vi "OutputShooter2.vi"() -> ()   [LabVIEW 2020]
uses:
  GRNF_CTREMotor.vi
  <vilib>/Rock Robotics/WPI/ThirdParty/Phoenix-LabVIEW/Motor Controller/Get/CTRE_Phoenix_MotorController_GetVoltage.vi
  <vilib>/Rock Robotics/WPI/ThirdParty/Phoenix-LabVIEW/Motor Controller/Get/CTRE_Phoenix_MotorController_GetSelectedSensorData.vi
  refnumbers.vi
  robotconstants.vi
  sensordata.vi
  robotoutputs.vi
  <vilib>/Rock Robotics/WPI/ThirdParty/Phoenix-LabVIEW/Motor Controller/Controls/CTRE_Phoenix_MotorControl_ControlMode.ctl
  TAI_Motor.vi
  98ea3fb8-6e38-4b27-9b09-ea0ebeb37837.vi
  driverdata.vi
  b8824af5-e744-4a1c-8f85-7ad47afccb2a.vi
  f2b47ff3-4a7b-451f-be46-1db9049ccf7f.vi
  drivercommands.vi
  <vilib>/Rock Robotics/WPI/ThirdParty/Phoenix-LabVIEW/Motor Controller/Get/CTRE_Phoenix_MotorController_GetGeneralStatus.vi
  176032df-062a-4c80-a46a-f01413ab376a.vi
  <vilib>/Rock Robotics/WPI/DriverStation/WPI_DriverStationRobotMode2.ctl
panel:
  in  "Shooter Upper PID Configuration":T1={"P Gain"=0.006, "I Gain"=0.0, "D Gain"=0.0, "F Gain"=0.2, "I Zone"=200.0} {"I Zone" step=0.01; "F Gain" step=0.01; "D Gain" step=0.01; "I Gain" step=0.01; "P Gain" min=0.0 step=0.01}
  in  "Cowl PID Parameters":T2={"Kp"=0.03, "Ki"=0.0, "Kd"=0.0, "Kf (don't use)"=0.0, "I-Zone"=10.0} {"Kd" min=0.0; "Ki" min=0.0; "Kp" min=0.0}
  in  "Arbitrary Feed Forward [-1,1]":dbl=0.03
  in  "Cowl S-Curve Strength":i32=4
  in  "Cowl Acceleration (deg/s^2)":dbl=300.0
  in  "Cowl Cruise Velocity (deg/s)":dbl=60.0
  out "Cowl Position":cluster{dbl, "Interlock Output":dbl}(graph)
  out "Position":dbl
  out "Cowl Velocity":cluster{dbl}(graph)
  in  "Plot Cowl":bool
  in  "Manual Override Cowl":bool
  in  "Manual Cowl Command (deg)":dbl
  in  "Manual Shooter Upper Speed Goal (rpm)":dbl=1.5 min=0.0 max=6000.0 step=100.0
  in  "Manual Shooter Lower Speed Goal (rpm)":dbl min=0.0 max=6000.0 step=100.0
  in  "Override Shooter State Controller":bool
  out "Shooter Upper":T3(graph)
  out "Shooter Lower":T3(graph)
  in  "Plot Shooter":bool
  in  "Shooter Lower PID Configuration":T1={"P Gain"=0.005, "I Gain"=0.0, "D Gain"=0.0, "F Gain"=0.2, "I Zone"=200.0} {"I Zone" step=0.01; "F Gain" step=0.01; "D Gain" step=0.01; "I Gain" step=0.01; "P Gain" min=0.0 step=0.01}
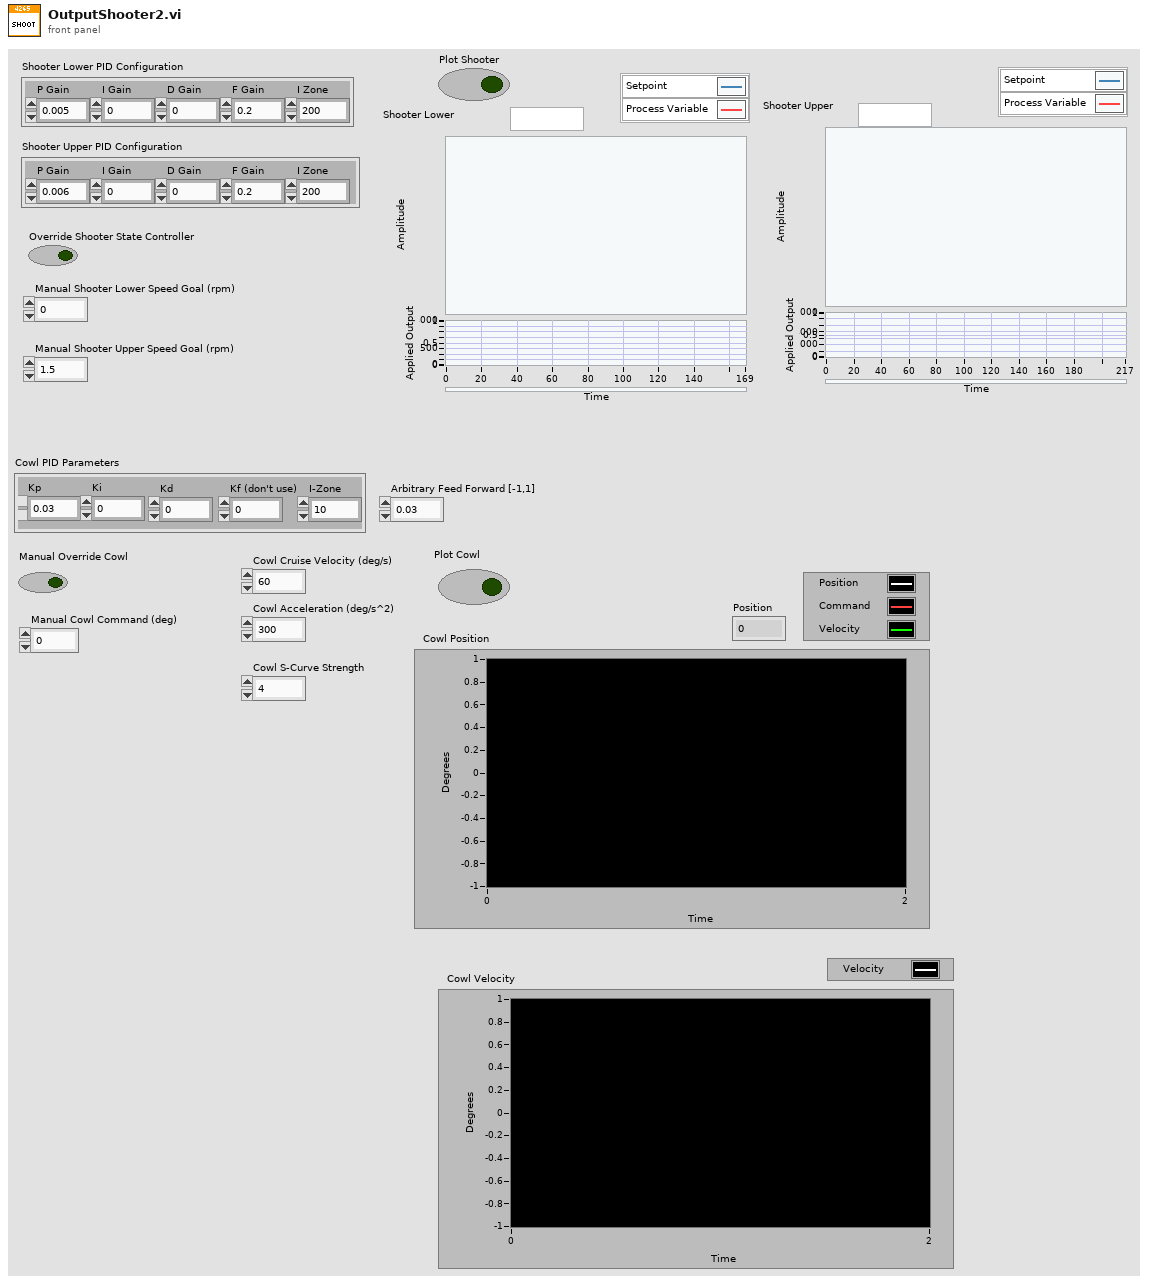
[diagram p1: front panel]
types:
  T1 = cluster{"P Gain":dbl, "I Gain":dbl, "D Gain":dbl, "F Gain":dbl, "I Zone":dbl}
  T2 = cluster{"Kp":dbl, "Ki":dbl, "Kd":dbl, "Kf (don't use)":dbl, "I-Zone":dbl}
  T3 = cluster{"Sensor Velocity":dbl, "Setpoint":dbl, "Applied Output":dbl}
  T4 = typedef "WPI_DriverStationRobotMode2.ctl" = enum16{"Autonomous Disabled", "Autonomous Enabled", "Teleop Disabled", "Teleop Enabled", "Disconnected", "Finish", "Test Disabled", "Test Enabled", "Emergency Stopped"}
  T5 = cluster{"Cowl Cruise Velocity (deg/s)":i32, "Cowl Acceleration (deg/s^2)":i32, "Cowl S-Curve Strength":i32}
  T6 = typedef "WPI_MotorControlDeviceRef.ctl" = cluster{"DeviceStatus":errorcluster, "Type":T7, "PWM":cluster{"PWM Channel":T8, "DeadBand":T9}, "CAN":cluster{"Device Number":u8, "SetOutput VI Ref":variant, "GetOutput VI Ref":variant, "Enable VI Ref":variant, "Disable VI Ref":variant, "Data":variant}, "Invert":bool, "DIO PWM":cluster{"PWM \"Enable\" Channel":T8, "DIOChannel":T10, "PWM Rate":dbl}}
  T7 = typedef "WPI_MotorControlType.ctl" = enum16{"PWM", "CAN", "DIO PWM"}
  T8 = typedef "FPGA_DIOPWMChannel.ctl" = enum8{"PWM 0", "PWM 1", "PWM 2", "PWM 3", "PWM 4", "PWM 5", "PWM 6", "PWM 7", "PWM 8", "PWM 9", "PWM MXP 0", "PWM MXP 1", "PWM MXP 2", "PWM MXP 3", "PWM MXP 4", "PWM MXP 5", "PWM MXP 6", "PWM MXP 7", "PWM MXP 8", "PWM MXP 9", "Invalid"}
  T9 = typedef "WPI_PWMDeadband.ctl" = cluster{"Name":string, "maxPositivePwm":i32, "minPositivePwm":i32, "centerPwm":i32, "maxNegativePwm":i32, "minNegativePwm":i32, "angularRange":u16}
  T10 = typedef "FPGA_DIOChannel.ctl" = enum8{"DIO 0", "DIO 1", "DIO 2", "DIO 3", "DIO 4", "DIO 5", "DIO 6", "DIO 7", "DIO 8", "DIO 9", "DIO MXP 0", "DIO MXP 1", "DIO MXP 2", "DIO MXP 3", "DIO MXP 4", "DIO MXP 5", "DIO MXP 6", "DIO MXP 7", "DIO MXP 8", "DIO MXP 9", "DIO MXP 10", "DIO MXP 11", "DIO MXP 12", "DIO MXP 13", "DIO MXP 14", "DIO MXP 15", "SPI Port CS1", "SPI Port CS2", "SPI Port CS3", "SPI Port MISO", "SPI Port MOSI", "Invalid"}
  T11 = cluster{"P Gain":bool, "I Gain":bool, "D Gain":bool, "F Gain":bool, "I Zone":bool}
  T12 = cluster{"Cowl Cruise Velocity (deg/s)":bool, "Cowl Acceleration (deg/s^2)":bool, "Cowl S-Curve Strength":bool}
  T13 = enum16{"No Changed Output", "New Normal Output", "New Testing Output"}
  T14 = cluster{"Kp":bool, "Ki":bool, "Kd":bool, "Kf (don't use)":bool, "I-Zone":bool}
  T15 = typedef "CTRE_Phoenix_MotorControl_ControlMode.ctl" = u16
  T16 = cluster{"Interlocked Output":dbl, dbl, "Percent Output":dbl}
  T17 = enum16{"DemandType_Neutral", "DemandType_AuxPID", "DemandType_ArbitraryFeedForward"}
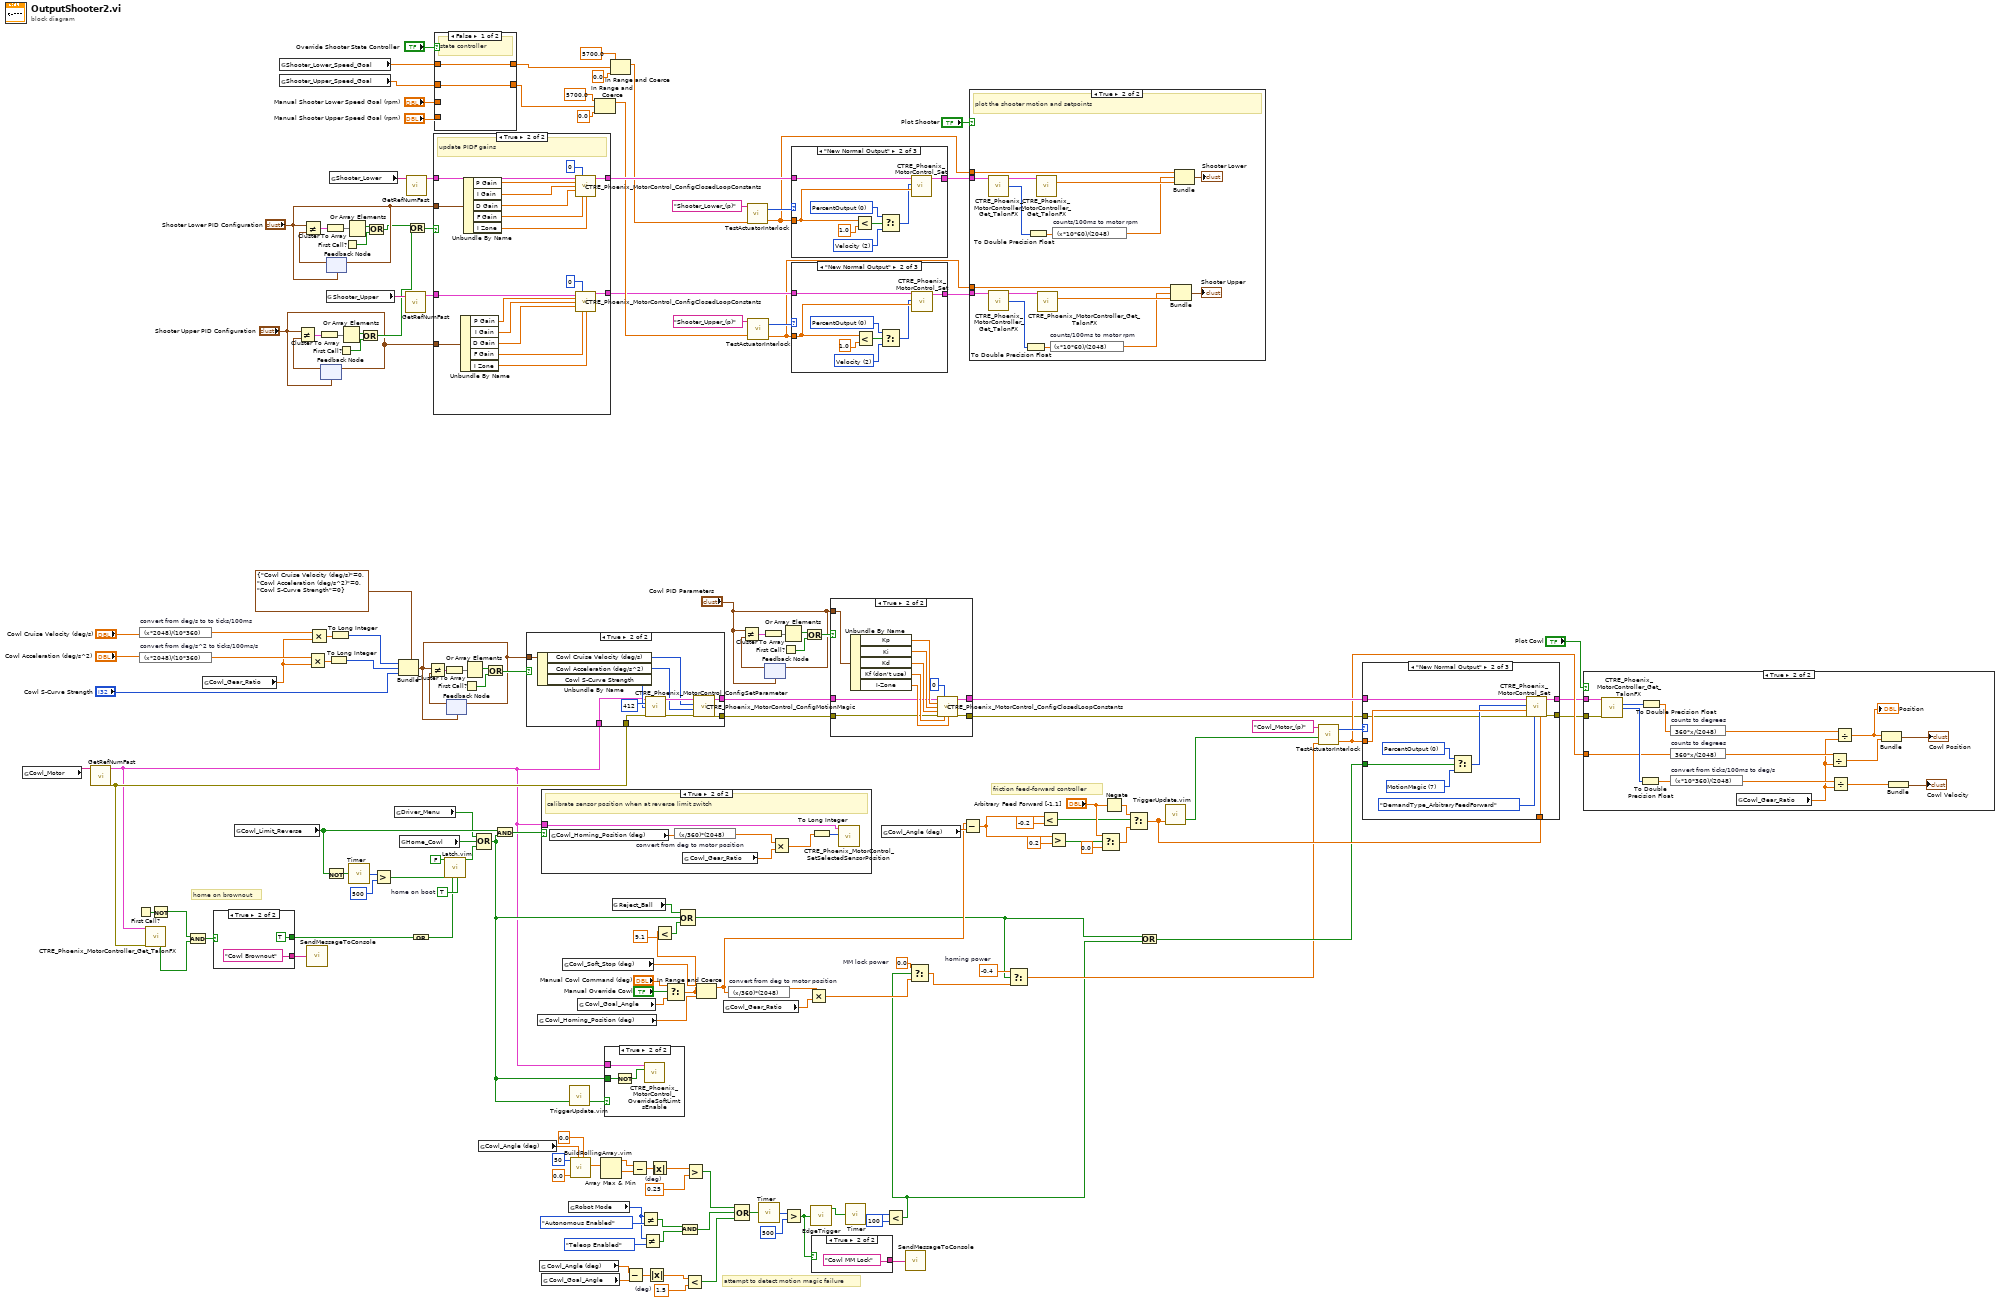
[diagram p0: block diagram]
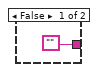
[diagram p2: hidden frame]
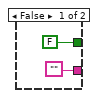
[diagram p3: hidden frame]
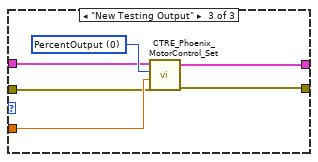
[diagram p6: hidden frame]
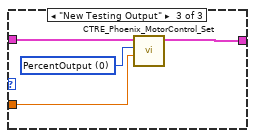
[diagram p8: hidden frame]
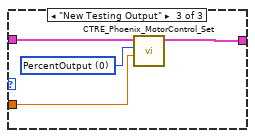
[diagram p10: hidden frame]
diagram:
  w9 = 0.0  # MM lock power
  w25 = 1.5  # (deg)
  w34 = 0.25  # (deg)
  w65 = TRUE  # home on boot
  w146 = -0.4  # homing power
  # "home on brownout"
  # "attempt to detect motion magic failure"
  # "friction feed-forward controller"
  n1 = global read "refnumbers.vi" "Cowl_Motor"() -> (w150:string)
  n2 = call-poly "GetRefNumFast.vi"("RefNum Name"=w150) -> ("Error"=w14:errorcluster, "Device Reference"=w13:T6)  [unwired: 5 in]
  n3 = First Call?() -> (First Call?: T/F=w45:bool)
  n4 = expression code="(x*2048)/(10*360)" "convert from deg/s to to ticks/100ms"("Cowl Cruise Velocity (deg/s)") -> (w98:dbl)
  n5 = expression code="(x*2048)/(10*360)" "convert from deg/s^2 to ticks/100ms/s"("Cowl Acceleration (deg/s^2)") -> (w99:dbl)
  n6 = call-poly <vilib>:"CTRE_Phoenix_MotorController_Get_TalonFX.vi"("PhoenixMotorControlDevRef"=w13, "error in"=w14) -> ("Has Reset Occurred?"=w47:bool)  [unwired: 8 in, 5 out]
  n7 = Not(x=w45) -> (.not. x?=w44:bool)
  n8 = And(x=w44, y=w47) -> (x .and. y?=w46:bool)
  n9 = global read "robotconstants.vi" "Cowl_Gear_Ratio"() -> (w97:dbl)
  n10 = case shown="True" w46 {
    tunnel: [FALSE TRUE] -> w12
    tunnel: ["" "Cowl Brownout" ("Message")] -> w17
    frame False {
    }
    frame True {
    }
  }
  n11 = global read "sensordata.vi" "Cowl_Limit_Reverse"() -> (w62:bool)
  n12 = global read "robotoutputs.vi" "Shooter_Lower_Speed_Goal"() -> (w129:dbl)
  n13 = global read "robotoutputs.vi" "Shooter_Upper_Speed_Goal"() -> (w128:dbl)
  n14 = call "SendMessageToConsole.vi"("Message String"=w17) -> ()  [unwired: 1 in]
  n15 = Multiply(x=w99, y=w97) -> (x*y=w100:dbl)
  n16 = Multiply(x=w98, y=w97) -> (x*y=w101:dbl)
  n17 = feedback #1("Shooter Upper PID Configuration") -> (w75:T1)
  n18 = Not Equal?(x="Shooter Upper PID Configuration", y=w75) -> (x != y?=w77:T11)
  n19 = Cluster To Array(cluster=w77) -> (array=w76:bool[])
  n20 = feedback-in #1("Shooter Upper PID Configuration") -> ()
  n21 = global read "refnumbers.vi" "Shooter_Upper"() -> (w154:string)
  n22 = Not(x=w62) -> (.not. x?=w64:bool)
  n23 = feedback #2("Shooter Lower PID Configuration") -> (w160:T1)
  n24 = Not Equal?(x="Shooter Lower PID Configuration", y=w160) -> (x != y?=w162:T11)
  n25 = Cluster To Array(cluster=w162) -> (array=w161:bool[])
  n26 = feedback-in #2("Shooter Lower PID Configuration") -> ()
  n27 = To Long Integer(number=w100) -> (32bit integer=w92:i32)
  n28 = global read "refnumbers.vi" "Shooter_Lower"() -> (w155:string)
  n29 = To Long Integer(number=w101) -> (32bit integer=w93:i32)
  n30 = First Call?() -> (First Call?: T/F=w79:bool)
  n31 = Or Array Elements(Boolean array=w76) -> (logical OR=w78:bool)
  n32 = First Call?() -> (First Call?: T/F=w164:bool)
  n33 = Or Array Elements(Boolean array=w161) -> (logical OR=w163:bool)
  n34 = call "Timer.vi"("Reset Timer"=w64) -> ("Time (ms)"=w68:u32)
  n35 = Or(x=w78, y=w79) -> (x .or. y?=w72:bool)
  n36 = Or(x=w163, y=w164) -> (x .or. y?=w73:bool)
  n37 = Greater?(x=w68, y=u32 500) -> (0:w63:bool)
  n38 = global read "drivercommands.vi" "Driver_Menu"() -> (w48:bool)
  n39 = Bundle(cluster=T5 {"Cowl Cruise Velocity (deg/s)"=0, "Cowl Acceleration (deg/s^2)"=0, "Cowl S-Curve Strength"=0}, "Cowl Cruise Velocity (deg/s)"=w93, "Cowl Acceleration (deg/s^2)"=w92, "Cowl S-Curve Strength"="Cowl S-Curve Strength") -> (w131:T5)
  n40 = global read "driverdata.vi" "Home_Cowl"() -> (w58:bool)
  n41 = call-poly "GetRefNumFast.vi"("RefNum Name"=w154) -> ("Device Reference"=w157:T6)  [unwired: 5 in, 1 out]
  n42 = call-poly "GetRefNumFast.vi"("RefNum Name"=w155) -> ("Device Reference"=w159:T6)  [unwired: 5 in, 1 out]
  n43 = Or(x=w73, y=w72) -> (x .or. y?=w74:bool)
  n44 = Compound Arithmetic op=OR(w12) -> (w54:bool)
  n45 = case shown="True" w74 {
    tunnel: w159 -> [w170 w187]
    tunnel: "Shooter Lower PID Configuration" -> [_ w186]
    tunnel: [w170 w188] -> w120
    tunnel: [w169 w185] -> w113
    tunnel: w157 -> [w169 w184]
    tunnel: "Shooter Upper PID Configuration" -> [_ w176]
    frame False {
      # "do not update PIDF gains"
    }
    frame True {
      # "update PIDF gains"
      n46 = Unbundle By Name(w176) -> ("P Gain"=w175:dbl, "I Gain"=w174:dbl, "D Gain"=w173:dbl, "F Gain"=w172:dbl, "I Zone"=w171:dbl)
      n47 = Unbundle By Name(w186) -> ("P Gain"=w183:dbl, "I Gain"=w182:dbl, "D Gain"=w181:dbl, "F Gain"=w177:dbl, "I Zone"=w180:dbl)
      n48 = call <vilib>:"CTRE_Phoenix_MotorControl_ConfigClosedLoopConstants.vi"("PhoenixMotorControlDevRef"=w187, "slotIdx"=0, "P"=w183, "I"=w182, "D"=w181, "F"=w177, "I Zone"=w180) -> ("PhoenixMotorControlDevRef"=w188:T6)  [unwired: 7 in, 1 out]
      n49 = call <vilib>:"CTRE_Phoenix_MotorControl_ConfigClosedLoopConstants.vi"("PhoenixMotorControlDevRef"=w184, "slotIdx"=0, "P"=w175, "I"=w174, "D"=w173, "F"=w172, "I Zone"=w171) -> ("PhoenixMotorControlDevRef"=w185:T6)  [unwired: 7 in, 1 out]
    }
  }
  n50 = case shown="False" "Override Shooter State Controller" {
    tunnel: "Manual Shooter Lower Speed Goal (rpm)" -> [_ w192]
    tunnel: "Manual Shooter Upper Speed Goal (rpm)" -> [_ w191]
    tunnel: w128 -> [w189 _]
    tunnel: w129 -> [w190 _]
    tunnel: [w190 w192] -> w125
    tunnel: [w189 w191] -> w1
    frame False {
      # "state controller"
    }
    frame True {
      # "manual control"
    }
  }
  n51 = call "Latch.vim"("Default Value"=w65, "Reset"=w54, "Latch Signal"=w63, "Latch Value"=FALSE) -> ("Latched"=w61:bool)  [unwired: 7 in]
  n52 = feedback #3(w131) -> (w132:T5)
  n53 = Not Equal?(x=w131, y=w132) -> (x != y?=w135:T12)
  n54 = Cluster To Array(cluster=w135) -> (array=w134:bool[])
  n55 = feedback-in #3(w131) -> ()
  n56 = First Call?() -> (First Call?: T/F=w137:bool)
  n57 = Or Array Elements(Boolean array=w134) -> (logical OR=w136:bool)
  n58 = Compound Arithmetic op=OR(w48, w58, w61) -> (w52:bool)
  n59 = global read "sensordata.vi" "Cowl_Angle (deg)"() -> (w43:dbl)
  n60 = Or(x=w136, y=w137) -> (x .or. y?=w133:bool)
  n61 = And(x=w62, y=w52) -> (x .and. y?=w59:bool)
  n62 = case shown="True" w133 {
    tunnel: w131 -> [_ w202]
    tunnel: w13 -> [w194 w198]
    tunnel: w14 -> [w193 w197]
    tunnel: [w194 w196] -> w110
    tunnel: [w193 w195] -> w109
    frame False {
    }
    frame True {
      n63 = Unbundle By Name(w202) -> ("Cowl Cruise Velocity (deg/s)"=w199:i32, "Cowl Acceleration (deg/s^2)"=w200:i32, "Cowl S-Curve Strength"=w201:i32)
      n64 = call <vilib>:"CTRE_Phoenix_MotorControl_ConfigSetParameter.vi"("PhoenixMotorControlDevRef"=w198, "Parameter"=412 ("New Sensor Position"), "value"=w201, "error in (no error)"=w197) -> ("PhoenixMotorControlDevRef"=w204:T6, "error out"=w203:errorcluster)  [unwired: 10 in]
      n65 = call <vilib>:"CTRE_Phoenix_MotorControl_ConfigMotionMagic.vi"("error in (no error)"=w203, "Acceleration"=w200, "Cruise Velocity"=w199, "PhoenixMotorControlDevRef"=w204) -> ("error out"=w195:errorcluster, "PhoenixMotorControlDevRef"=w196:T6)  [unwired: 6 in]
    }
  }
  n66 = global read "robotconstants.vi" "Cowl_Homing_Position (deg)"() -> (w55:dbl)
  n67 = global read "sensordata.vi" "Cowl_Angle (deg)"() -> (w27:dbl)
  n68 = case shown="True" w59 {
    tunnel: w13 -> [_ w210]
    frame False {
    }
    frame True {
      # "calibrate sensor position when at reverse limit switch"
      n69 = global read "robotconstants.vi" "Cowl_Homing_Position (deg)"() -> (w209:dbl)
      n70 = expression code="(x/360)*(2048)" "convert from deg to motor position"(w209) -> (w207:dbl)
      n71 = global read "robotconstants.vi" "Cowl_Gear_Ratio"() -> (w208:dbl)
      n72 = Multiply(x=w207, y=w208) -> (x*y=w206:dbl)
      n73 = To Long Integer(number=w206) -> (32bit integer=w211:i32)
      n74 = call <vilib>:"CTRE_Phoenix_MotorControl_SetSelectedSensorPosition.vi"("New Sensor Position"=w211, "PhoenixMotorControlDevRef"=w210) -> ()  [unwired: 8 in, 2 out]
    }
  }
  n75 = global read "robotoutputs.vi" "Cowl_Goal_Angle"() -> (w28:dbl)
  n76 = global read "robotconstants.vi" "Cowl_Soft_Stop (deg)"() -> (w81:dbl)
  n77 = global read "driverdata.vi" "Robot Mode"() -> (w31:T4)
  n78 = call "TriggerUpdate.vim"("Trigger"=w52) -> ("Update"=w53:bool)  [unwired: 2 in]
  n79 = call "BuildRollingArray.vim"("Global Additive Update"=0.0, "New Value"=w43, "Initial Value"=0.0, "Number of Elements"=50) -> ("Current Array"=w39:dbl[])  [unwired: 7 in]
  n80 = global read "robotoutputs.vi" "Cowl_Goal_Angle"() -> (w130:dbl)
  n81 = In Range and Coerce(upper limit=5700.0, x=w1, lower limit=0.0) -> (coerced(x)=w114:dbl)  [unwired: 1 out]
  n82 = Array Max & Min(array=w39) -> (max value=w38:dbl, min value=w37:dbl)  [unwired: 2 out]
  n83 = case shown="True" w53 {
    tunnel: w52 -> [_ w214]
    tunnel: w13 -> [_ w212]
    frame False {
    }
    frame True {
      n84 = Not(x=w214) -> (.not. x?=w213:bool)
      n85 = call <vilib>:"CTRE_Phoenix_MotorControl_OverrideSoftLimtsEnable.vi"("PhoenixMotorControlDevRef"=w212, "Override Soft Limit Enable?"=w213) -> ()  [unwired: 12 in, 2 out]
    }
  }
  n86 = In Range and Coerce(upper limit=5700.0, x=w125, lower limit=0.0) -> (coerced(x)=w119:dbl)  [unwired: 1 out]
  n87 = global read "robotoutputs.vi" "Reject_Ball"() -> (w60:bool)
  n88 = Subtract(x=w27, y=w28) -> (x-y=w26:dbl)
  n89 = Subtract(x=w38, y=w37) -> (x-y=w36:dbl)
  n90 = Not Equal?(x=w31, y=WPI_DriverStationRobotMode2."Autonomous Enabled") -> (x != y?=w30:bool)
  n91 = Not Equal?(x=w31, y=WPI_DriverStationRobotMode2."Teleop Enabled") -> (x != y?=w29:bool)
  n92 = Absolute Value(x=w26) -> (abs(x)=w24:dbl)
  n93 = Absolute Value(x=w36) -> (abs(x)=w35:dbl)
  n94 = Select(t="Manual Cowl Command (deg)", s="Manual Override Cowl", f=w130) -> (s? t:f=w50:dbl)
  n95 = Less?(x=w50, y=9.1) -> (x < y?=w51:bool)
  n96 = Compound Arithmetic op=OR(w60, w52, w51) -> (w11:bool)
  n97 = Compound Arithmetic op=AND(w30, w29) -> (w20:bool)
  n98 = Less?(x=w24, y=w25) -> (x < y?=w19:bool)
  n99 = Greater?(x=w35, y=w34) -> (0:w21:bool)
  n100 = In Range and Coerce(upper limit=w81, x=w50, lower limit=w55) -> (coerced(x)=w80:dbl)  [unwired: 1 out]
  n101 = global read "robotconstants.vi" "Cowl_Gear_Ratio"() -> (w103:dbl)
  n102 = expression code="(x/360)*(2048)" "convert from deg to motor position"(w80) -> (w102:dbl)
  n103 = Compound Arithmetic op=OR(w21, w20, w19) -> (w18:bool)
  n104 = call-poly "TestActuatorInterlock.vi"("Normal Output"=w119, "Actuator Name"="Shooter_Lower_(p)" ("Actuator_Name")) -> ("Interlocked Output"=w118:dbl, "Output Mode"=w122:T13)  [unwired: 3 in]
  n105 = call-poly "TestActuatorInterlock.vi"("Normal Output"=w114, "Actuator Name"="Shooter_Upper_(p)" ("Actuator_Name")) -> ("Interlocked Output"=w111:dbl, "Output Mode"=w116:T13)  [unwired: 3 in]
  n106 = call "Timer.vi"("Reset Timer"=w18) -> ("Time (ms)"=w22:u32)
  n107 = feedback #4("Cowl PID Parameters") -> (w140:T2)
  n108 = Not Equal?(x="Cowl PID Parameters", y=w140) -> (x != y?=w143:T14)
  n109 = Cluster To Array(cluster=w143) -> (array=w142:bool[])
  n110 = feedback-in #4("Cowl PID Parameters") -> ()
  n111 = First Call?() -> (First Call?: T/F=w145:bool)
  n112 = Or Array Elements(Boolean array=w142) -> (logical OR=w144:bool)
  n113 = Greater?(x=w22, y=u32 500) -> (0:w15:bool)
  n114 = case shown="\"New Normal Output\"" w122 {
    tunnel: w120 -> [w215 w223 w226]
    tunnel: w118 -> [_ w218 w225]
    tunnel: [w215 w222 w224] -> w117
    frame "No Changed Output", Default {
    }
    frame "New Normal Output" {
      w220 = T15 0 items=["PercentOutput"=0, "Position"=1, "Velocity"=2, "Current"=3, "Follower"=5, "MotionProfile"=6, "MotionMagic"=7, "MotionProfileArc"=10, "Disabled"=15] ("Control Mode")
      w221 = T15 2 items=["PercentOutput"=0, "Position"=1, "Velocity"=2, "Current"=3, "Follower"=5, "MotionProfile"=6, "MotionMagic"=7, "MotionProfileArc"=10, "Disabled"=15] ("Control Mode")
      n115 = Less?(x=w218, y=1.0) -> (x < y?=w217:bool)
      n116 = Select(t=w220, s=w217, f=w221) -> (s? t:f=w216:T15)
      n117 = call <vilib>:"CTRE_Phoenix_MotorControl_Set.vi"("Output"=w218, "Control Mode"=w216, "PhoenixMotorControlDevRef"=w223) -> ("PhoenixMotorControlDevRef"=w222:T6)  [unwired: 7 in, 1 out]
    }
    frame "New Testing Output" {
      w227 = T15 0 items=["PercentOutput"=0, "Position"=1, "Velocity"=2, "Current"=3, "Follower"=5, "MotionProfile"=6, "MotionMagic"=7, "MotionProfileArc"=10, "Disabled"=15] ("Control Mode")
      n118 = call <vilib>:"CTRE_Phoenix_MotorControl_Set.vi"("Output"=w225, "Control Mode"=w227, "PhoenixMotorControlDevRef"=w226) -> ("PhoenixMotorControlDevRef"=w224:T6)  [unwired: 7 in, 1 out]
    }
  }
  n119 = case shown="\"New Normal Output\"" w116 {
    tunnel: w113 -> [w228 w236 w239]
    tunnel: w111 -> [_ w231 w238]
    tunnel: [w228 w235 w237] -> w112
    frame "No Changed Output", Default {
    }
    frame "New Normal Output" {
      w233 = T15 0 items=["PercentOutput"=0, "Position"=1, "Velocity"=2, "Current"=3, "Follower"=5, "MotionProfile"=6, "MotionMagic"=7, "MotionProfileArc"=10, "Disabled"=15] ("Control Mode")
      w234 = T15 2 items=["PercentOutput"=0, "Position"=1, "Velocity"=2, "Current"=3, "Follower"=5, "MotionProfile"=6, "MotionMagic"=7, "MotionProfileArc"=10, "Disabled"=15] ("Control Mode")
      n120 = Less?(x=w231, y=1.0) -> (x < y?=w230:bool)
      n121 = Select(t=w233, s=w230, f=w234) -> (s? t:f=w229:T15)
      n122 = call <vilib>:"CTRE_Phoenix_MotorControl_Set.vi"("Output"=w231, "Control Mode"=w229, "PhoenixMotorControlDevRef"=w236) -> ("PhoenixMotorControlDevRef"=w235:T6)  [unwired: 7 in, 1 out]
    }
    frame "New Testing Output" {
      w240 = T15 0 items=["PercentOutput"=0, "Position"=1, "Velocity"=2, "Current"=3, "Follower"=5, "MotionProfile"=6, "MotionMagic"=7, "MotionProfileArc"=10, "Disabled"=15] ("Control Mode")
      n123 = call <vilib>:"CTRE_Phoenix_MotorControl_Set.vi"("Output"=w238, "Control Mode"=w240, "PhoenixMotorControlDevRef"=w239) -> ("PhoenixMotorControlDevRef"=w237:T6)  [unwired: 7 in, 1 out]
    }
  }
  n124 = Or(x=w144, y=w145) -> (x .or. y?=w141:bool)
  n125 = Multiply(x=w102, y=w103) -> (x*y=w5:dbl)
  n126 = call "EdgeTrigger.vi"("Input Signal"=w15) -> ("Rising Edge Trigger"=w6:bool)  [unwired: 2 out]
  n127 = case shown="True" w15 {
    tunnel: ["" "Cowl MM Lock" ("Message")] -> w16
    frame False {
    }
    frame True {
    }
  }
  n128 = case shown="True" w141 {
    tunnel: "Cowl PID Parameters" -> [_ w251]
    tunnel: w110 -> [w244 w248]
    tunnel: w109 -> [w243 w247]
    tunnel: [w244 w246] -> w106
    tunnel: [w243 w245] -> w104
    frame False {
    }
    frame True {
      n129 = Unbundle By Name(w251) -> ("Kp"=w253:dbl, "Ki"=w254:dbl, "Kd"=w255:dbl, "Kf (don't use)"=w250:dbl, "I-Zone"=w249:dbl)
      n130 = call <vilib>:"CTRE_Phoenix_MotorControl_ConfigClosedLoopConstants.vi"("PhoenixMotorControlDevRef"=w248, "slotIdx"=0, "P"=w253, "I"=w254, "D"=w255, "error in (no error)"=w247, "F"=w250, "I Zone"=w249) -> ("PhoenixMotorControlDevRef"=w246:T6, "error out"=w245:errorcluster)  [unwired: 6 in]
    }
  }
  n131 = call "Timer.vi"("Reset Timer"=w6) -> ("Time (ms)"=w8:u32)
  n132 = global read "sensordata.vi" "Cowl_Angle (deg)"() -> (w91:dbl)
  n133 = Less?(x=w8, y=u32 100) -> (x < y?=w2:bool)
  n134 = call "SendMessageToConsole.vi"("Message String"=w16) -> ()  [unwired: 1 in]
  n135 = Select(t=w9, s=w2, f=w5) -> (s? t:f=w4:dbl)
  n136 = Subtract(x=w80, y=w91) -> (x-y=w85:dbl)
  n137 = case shown="True" "Plot Shooter" {
    tunnel: w118 -> [_ w271]
    tunnel: w117 -> [_ w267]
    tunnel: w112 -> [_ w266]
    tunnel: w111 -> [_ w264]
    frame False {
      # "disable plotting and expensive sensor polling"
    }
    frame True {
      # "plot the shooter motion and setpoints"
      n138 = call-poly <vilib>:"CTRE_Phoenix_MotorController_Get_TalonFX.vi"("PhoenixMotorControlDevRef"=w267) -> ("PhoenixMotorControlDevRef"=w268:T6, "Velocity (Raw Sensor Units per 100 ms)"=w262:i32)  [unwired: 11 in, 2 out]
      n139 = call-poly <vilib>:"CTRE_Phoenix_MotorController_Get_TalonFX.vi"("PhoenixMotorControlDevRef"=w266) -> ("PhoenixMotorControlDevRef"=w265:T6, "Velocity (Raw Sensor Units per 100 ms)"=w257:i32)  [unwired: 11 in, 2 out]
      n140 = To Double Precision Float(number=w257) -> (double precision float=w258:dbl)
      n141 = To Double Precision Float(number=w262) -> (double precision float=w263:dbl)
      n142 = call-poly <vilib>:"CTRE_Phoenix_MotorController_Get_TalonFX.vi"("PhoenixMotorControlDevRef"=w268) -> ("Percent Output"=w269:dbl)  [unwired: 10 in, 4 out]
      n143 = call-poly <vilib>:"CTRE_Phoenix_MotorController_Get_TalonFX.vi"("PhoenixMotorControlDevRef"=w265) -> ("Percent Output"=w270:dbl)  [unwired: 10 in, 4 out]
      n144 = expression code="(x*10*60)/(2048)" "counts/100ms to motor rpm"(w258) -> (w256:dbl)
      n145 = expression code="(x*10*60)/(2048)" "counts/100ms to motor rpm"(w263) -> (w261:dbl)
      n146 = Bundle("Interlocked Output"=w264, w256, "Percent Output"=w270) -> (→"Shooter Upper":T16)  [unwired: 1 in]
      n147 = Bundle("Interlocked Output"=w271, w261, "Percent Output"=w269) -> (→"Shooter Lower":T16)  [unwired: 1 in]
    }
  }
  n148 = Select(t=w146, s=w11, f=w4) -> (s? t:f=w3:dbl)
  n149 = Less?(x=w85, y=-0.2) -> (x < y?=w82:bool)
  n150 = Greater?(x=w85, y=0.2) -> (0:w90:bool)
  n151 = Select(t="Arbitrary Feed Forward [-1,1]", s=w90, f=0.0) -> (s? t:f=w89:dbl)
  n152 = Negate(x="Arbitrary Feed Forward [-1,1]") -> (-x=w88:dbl)
  n153 = Select(t=w88, s=w82, f=w89) -> (s? t:f=w69:dbl)
  n154 = Or(x=w11, y=w2) -> (x .or. y?=w10:bool)
  n155 = call "TriggerUpdate.vim"("Trigger"=w69) -> ("Update"=w70:bool)  [unwired: 2 in]
  n156 = call-poly "TestActuatorInterlock.vi"("Normal Output"=w3, "Aux Trigger"=w70, "Actuator Name"="Cowl_Motor_(p)" ("Actuator_Name")) -> ("Interlocked Output"=w105:dbl, "Output Mode"=w108:T13)  [unwired: 2 in]
  n157 = case shown="\"New Normal Output\"" w108 {
    tunnel: w106 -> [w273 w284 w289]
    tunnel: w105 -> [_ w280 w288]
    tunnel: [w273 w283 w287] -> w57
    tunnel: w10 -> [_ w278 _]
    tunnel: w69 -> [_ w276 _]
    tunnel: [w272 w275 w285] -> w56
    tunnel: w104 -> [w272 w274 w286]
    frame "No Changed Output", Default {
    }
    frame "New Normal Output" {
      w281 = T15 0 items=["PercentOutput"=0, "Position"=1, "Velocity"=2, "Current"=3, "Follower"=5, "MotionProfile"=6, "MotionMagic"=7, "MotionProfileArc"=10, "Disabled"=15] ("Control Mode")
      w282 = T15 7 items=["PercentOutput"=0, "Position"=1, "Velocity"=2, "Current"=3, "Follower"=5, "MotionProfile"=6, "MotionMagic"=7, "MotionProfileArc"=10, "Disabled"=15] ("Control Mode")
      n158 = Select(t=w281, s=w278, f=w282) -> (s? t:f=w279:T15)
      n159 = call <vilib>:"CTRE_Phoenix_MotorControl_Set.vi"("Demand1"=w276, "DemandType"=T17."DemandType_ArbitraryFeedForward", "error in (no error)"=w274, "Output"=w280, "Control Mode"=w279, "PhoenixMotorControlDevRef"=w284) -> ("error out"=w275:errorcluster, "PhoenixMotorControlDevRef"=w283:T6)  [unwired: 4 in]
    }
    frame "New Testing Output" {
      w290 = T15 0 items=["PercentOutput"=0, "Position"=1, "Velocity"=2, "Current"=3, "Follower"=5, "MotionProfile"=6, "MotionMagic"=7, "MotionProfileArc"=10, "Disabled"=15] ("Control Mode")
      n160 = call <vilib>:"CTRE_Phoenix_MotorControl_Set.vi"("error in (no error)"=w286, "Output"=w288, "Control Mode"=w290, "PhoenixMotorControlDevRef"=w289) -> ("error out"=w285:errorcluster, "PhoenixMotorControlDevRef"=w287:T6)  [unwired: 6 in]
    }
  }
  n161 = case shown="True" "Plot Cowl" {
    tunnel: w105 -> [_ w299]
    tunnel: w56 -> [_ w302]
    tunnel: w57 -> [_ w301]
    frame False {
    }
    frame True {
      n162 = call-poly <vilib>:"CTRE_Phoenix_MotorController_Get_TalonFX.vi"("PhoenixMotorControlDevRef"=w301, "error in"=w302) -> ("Position (Raw Sensor Units)"=w304:i32, "Velocity (Raw Sensor Units per 100 ms)"=w305:i32)  [unwired: 10 in, 2 out]
      n163 = To Double Precision Float(number=w305) -> (double precision float=w306:dbl)
      n164 = To Double Precision Float(number=w304) -> (double precision float=w303:dbl)
      n165 = expression code="360*x/(2048)" "counts to degrees"(w303) -> (w292:dbl)
      n166 = expression code="360*x/(2048)" "counts to degrees"(w299) -> (w295:dbl)
      n167 = expression code="(x*10*360)/(2048)" "convert from ticks/100ms to deg/s"(w306) -> (w297:dbl)
      n168 = global read "robotconstants.vi" "Cowl_Gear_Ratio"() -> (w293:dbl)
      n169 = Divide(x=w295, y=w293) -> (x/y=w294:dbl)
      n170 = Divide(x=w297, y=w293) -> (x/y=w296:dbl)
      n171 = Divide(x=w292, y=w293) -> (x/y=w291:dbl)
      "Position" <- w291
      n172 = Bundle(w291, w294) -> (→"Cowl Position":cluster{dbl, dbl})  [unwired: 1 in]
      n173 = Bundle(w296) -> (→"Cowl Velocity":cluster{dbl})  [unwired: 1 in]
    }
  }
